vi "VariableWriteUIAsync.vi"(10 "VariableFill":refnum<class "Variable.lvclass">, 11 "VariableManagerRef in":refnum<vi>) -> ()   [LabVIEW 2013]
doc: "Asynchronously call VariableWriteUI.vi with the given input. The caller process will not be blocked."
uses:
  VariableManager/VariableManager.lvclass
  Variable/Variable.lvclass
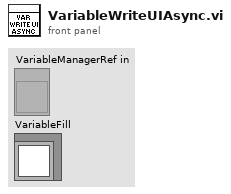
[diagram p1: front panel]
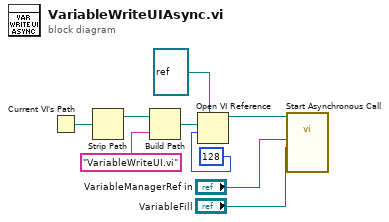
[diagram p0: block diagram]
diagram:
  n1 = Current VI's Path() -> (path=w7:path)
  n2 = Strip Path(path=w7) -> (stripped path=w8:path)  [unwired: 1 out]
  n3 = Build Path(base path=w8, name or relative path="VariableWriteUI.vi") -> (appended path=w6:path)
  n4 = Open VI Reference(type specifier VI Refnum (for type only)=refnum<vi> refnum, vi path=w6, options=128) -> (vi reference=w4:refnum<vi>)  [unwired: 3 in, 1 out]
  n5 = call-by-ref "Start Asynchronous Call"(reference=w4, "VariableFill"="VariableFill", "VariableManagerRef in"="VariableManagerRef in") -> ()  [unwired: 9 in, 4 out]
